vi "Expression Array String to Expression Array.vi"(11 "Expression Array String":string) -> (3 "Expression Array":string[](array[string]))   [LabVIEW 2013, in "RTSequenceVIs.lvlib"]
doc: "Takes an expression array string in the form of {X,Y,Z} and converts it into an array of strings."
uses:
  RTSequenceVIs.lvlib
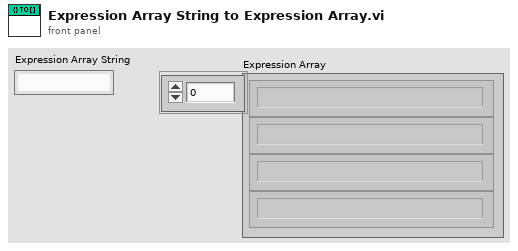
[diagram p1: front panel]
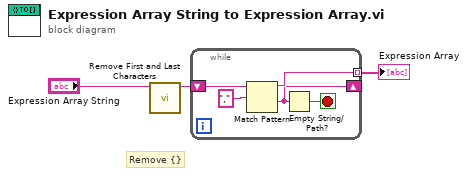
[diagram p0: block diagram]
diagram:
  # "Remove {}"
  n1 = call "Remove First and Last Characters.vi"("Quoted String"="Expression Array String") -> ("String"=w2:string)  [unwired: 10 in]
  n2 = while {
    shift-right: [w4] -> _
    shift-left: w2 -> [w7]
    tunnel: [w5] -> w3 mode=indexing
    stop <- w8 stop-if-true
    n3 = Match Pattern(string=w7, regular expression="," ("search string/char (-)")) -> (before substring=w5:string, after substring=w4:string)  [unwired: 1 in, 2 out]
    n4 = Empty String/Path?(string/path=w4) -> (empty?=w8:bool)
  }
  "Expression Array" <- w3
